vi "Autonomous Independent.vi"() -> ()   [LabVIEW 2016]
doc: "This VI is called when autonomous begins, and will automatically be terminated when autonomous ends. You can carry out timed or sensor driven robot movement independently without needing to return to the caller."
uses:
  <vilib>/Rock Robotics/WPI/Solenoid/WPI_SolenoidValue.ctl
  <vilib>/Rock Robotics/WPI/Utilities/WPI_GetSetVariantRefNum.vi
  <vilib>/Rock Robotics/Network Tables/NT Read String.vi
  <vilib>/Rock Robotics/Network Tables/NT Write Numeric Array.vi
  <vilib>/Rock Robotics/WPI/Solenoid/WPI_SolenoidSetEnum.vi
  SubSystems/Drive/Drive System.lvlib
  SubSystems/Intake/Intake.lvlib
  Vision/Vision Drive/Vision Drive.lvlib
  SubSystems/Path Track/Path Track.lvlib
panel:
  in  "Gear Auton Settings":T1(tab)=enum."Boiler Side Auton"
  in  "Center Gear Distance":dbl=81.0
  in  "First Turn Angle Hopper":dbl=60.0 caption="First Turn Angle"
  in  "First Drive Distance Hopper":dbl=95.0 caption="First Drive Distance"
  in  "Second Drive Distance Hopper":dbl=53.0 caption="Second Drive Distance"
  in  "Second Drive Distance":dbl=53.0
  in  "First Turn Angle":dbl=-60.0
  in  "First Drive Distance":dbl=95.0
  out "Distance (in) 2":dbl
  in  "Angle 2":dbl=30.0 format="%#_13g"
  in  "Distance (in)":dbl=-120.0 format="%#_13g"
  # "Distances:\n\n93.25\" to alignment line\n114.3\" to front of airship"
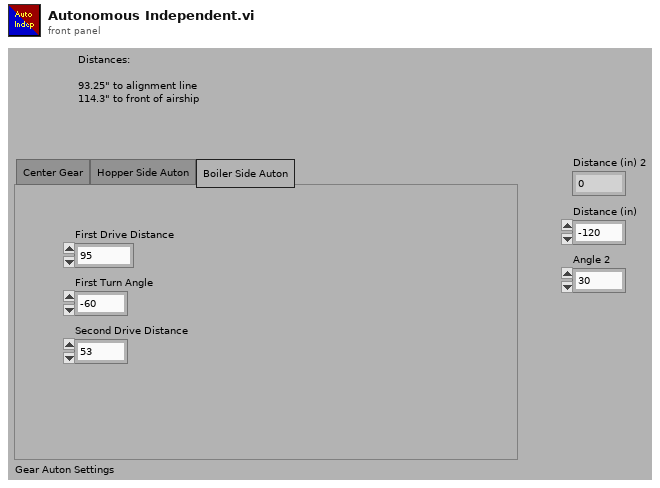
[diagram p1: front panel]
types:
  T1 = enum32{"Center Gear", "Hopper Side Auton", "Boiler Side Auton"}
  T2 = typedef "WPI_SolenoidValue.ctl" = enum16{"Off", "On", "Forward", "Reverse"}
  T3 = typedef "WPI_JoystickDevRef.ctl" = cluster{"Device":T4}
  T4 = typedef "WPI_JoystickDeviceEnum.ctl" = enum16{"USB 0", "USB 1", "USB 2", "USB 3", "USB 4", "USB 5"}
  T5 = typedef "WPI_SolenoidDevRef.ctl" = cluster{"DevStatus":errorcluster, "Pneumatics Control Module":u8, "Forward Solenoid Channel":T6, "Reverse Solenoid Channel":T6}
  T6 = typedef "WPI_SolenoidChannel.ctl" = enum8{"Solenoid 0", "Solenoid 1", "Solenoid 2", "Solenoid 3", "Solenoid 4", "Solenoid 5", "Solenoid 6", "Solenoid 7", "Invalid"}
  T7 = enum16{"Do Nothing", "Turn Up Field", "Turn to Boiler"}
  T8 = typedef "WPI_GyroDevRef.ctl" = cluster{"DevStatus":errorcluster, "Analog Channel":T9, "Offset":dbl, "Gain (VoltsPerDegree/Second)":dbl, "Gyro Type":enum16{"Analog", "XRS450"}, "Handle":i32, "SPI Bus":T10, "Device Found":bool, "Sample Rate":dbl, "Calibrate On Open":bool}
  T9 = typedef "FPGA_AIChannel.ctl" = enum8{"AI 0", "AI 1", "AI 2", "AI 3", "AI MXP 0", "AI MXP 1", "AI MXP 2", "AI MXP 3", "Invalid"}
  T10 = typedef "spi_bus.ctl" = enum16{"SPI On-Board, CS0", "SPI On-Board, CS1", "SPI On-Board, CS2", "SPI On-Board, CS3", "SPI MXP", "Invalid"}
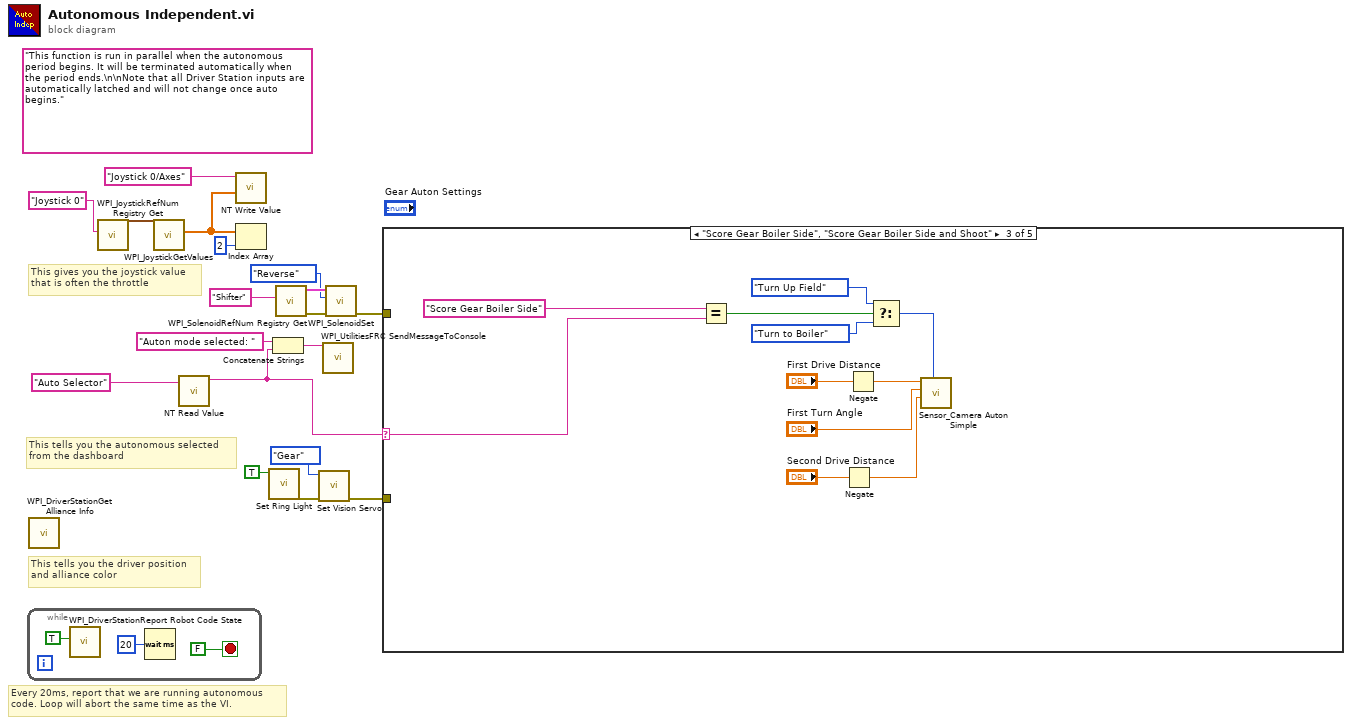
[diagram p0: block diagram]
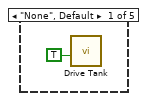
[diagram p2: hidden frame]
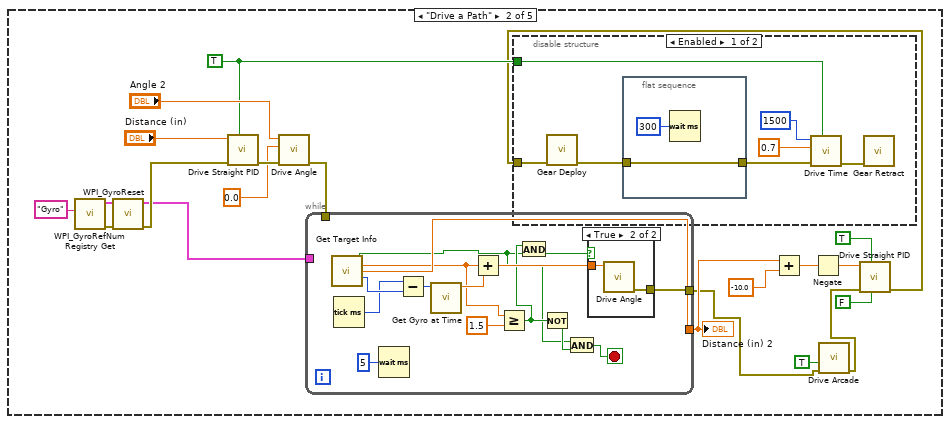
[diagram p3: hidden frame]
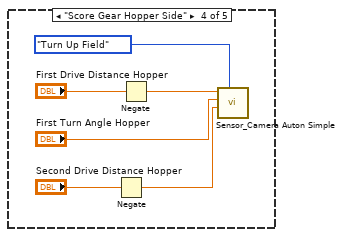
[diagram p6: hidden frame]
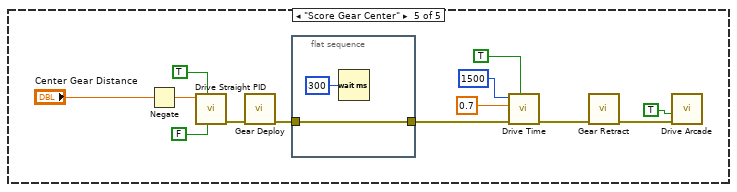
[diagram p7: hidden frame]
diagram:
  (unwired) "This function is run in parallel when the autonomous period begins. It will be terminated automatically when the period ends.\n\nNote that all Driver Station inputs are automatically latched and will not change once auto begins."
  # "This tells you the autonomous selected\nfrom the dashboard"
  # "Every 20ms, report that we are running autonomous\ncode. Loop will abort the same time as the VI."
  # "This gives you the joystick value\nthat is often the throttle"
  # "This tells you the driver position\nand alliance color"
  n1 = while {
    stop <- FALSE stop-if-true
    n2 = call <vilib>:"WPI_DriverStationReport Robot Code State.vi"("Autonomous"=TRUE) -> ()  [unwired: 10 in, 1 out]
    n3 = Wait (ms)(milliseconds to wait=u32 20) -> ()  [unwired: 1 out]
  }
  n4 = call <vilib>:"WPI_DriverStationGet Alliance Info.vi"() -> ()  [unwired: 12 out]
  n5 = call <vilib>:"WPI_JoystickRefNum Registry Get.vi"("refnum name"="Joystick 0") -> ("JoystickDevRef"=w17:T3)  [unwired: 1 in, 9 out]
  n6 = call <vilib>:"WPI_JoystickGetValues.vi"("JoystickDevRef"=w17) -> ("Axes"=w14:dbl[])  [unwired: 6 in, 4 out]
  n7 = call-poly <vilib>:"NT Read Value.vi"("Name"="Auto Selector") -> ("String"=w10:string)  [unwired: 9 in, 1 out]
  n8 = call-poly <vilib>:"NT Write Value.vi"("Numeric Array"=w14, "Name"="Joystick 0/Axes") -> ()  [unwired: 9 in, 1 out]
  n9 = Index Array(array=w14, index=2) -> ()  [unwired: 1 out]
  n10 = call "Set Ring Light.vi"("Light On? (F)"=TRUE) -> ("error out"=w7:errorcluster)  [unwired: 10 in]
  n11 = Concatenate Strings("Auton mode selected: " ("string"), w10) -> (w11:string)
  n12 = call <vilib>:"WPI_SolenoidRefNum Registry Get.vi"("refnum name"="Shifter") -> ("error out"=w4:errorcluster, "SolenoidDevRef"=w3:T5)  [unwired: 9 in]
  n13 = call "Set Vision Servo.vi"("error in"=w7, "Setting"=enum16{"Custom", "Boiler", "Gear"}."Gear") -> ("error out"=w6:errorcluster)  [unwired: 9 in]
  n14 = call <vilib>:"WPI_UtilitiesFRC SendMessageToConsole.vi"("Message"=w11) -> ()  [unwired: 14 in, 1 out]
  n15 = call-poly <vilib>:"WPI_SolenoidSet.vi"("error in (no error)"=w4, "Value"=WPI_SolenoidValue."Reverse", "SolenoidDevRef"=w3) -> ("error out"=w1:errorcluster)  [unwired: 7 in, 1 out]
  n16 = case shown="\"Score Gear Boiler Side\", \"Score Gear Boiler Side and Shoot\"" w10 {
    selector: w10 -> [_ _ w76 _ _]
    tunnel: w6 -> [_ _ _ _ _]
    tunnel: w1 -> [_ _ _ _ _]
    frame "None", Default {
      n17 = call "Drive Tank.vi"("Force? (F)"=TRUE) -> ()  [unwired: 10 in, 1 out]
    }
    frame "Drive a Path" {
      w41 = TRUE ("Wait for Completion? (F)")
      n18 = call <vilib>:"WPI_GyroRefNum Registry Get.vi"("refnum name"="Gyro") -> ("error out"=w39:errorcluster, "GyroDevRef"=w38:T8)  [unwired: 9 in]
      n19 = call <vilib>:"WPI_GyroReset.vi"("error in"=w39, "GyroDevRef"=w38) -> ("error out"=w36:errorcluster, "GyroDevRef"=w34:T8)  [unwired: 8 in]
      n20 = call "Drive Straight PID.vi"("Wait for Completion? (F)"=w41, "error in"=w36, "Distance (in)"="Distance (in)") -> ("error out"=w43:errorcluster)  [unwired: 8 in]
      n21 = call "Drive Angle.vi"("error in"=w43, "Drive Magnitude"=0.0, "Angle"="Angle 2") -> ("error out"=w35:errorcluster)  [unwired: 8 in]
      n22 = while {
        tunnel: w35 -> [_]
        tunnel: w34 -> [_]
        tunnel: [w52] -> w32
        tunnel: [w47] -> w26
        stop <- w49 stop-if-true
        n23 = call "Get Target Info.vi"() -> ("Target Found?"=w48:bool, "Angle (deg)"=w51:dbl, "Distance (in)"=w52:dbl, "timestamp"=w46:u32)  [unwired: 11 in, 1 out]
        n24 = Tick Count (ms)() -> (millisecond timer value=w44:u32)
        n25 = Wait (ms)(milliseconds to wait=u32 5) -> ()  [unwired: 1 out]
        n26 = Subtract(x=w44, y=w46) -> (x-y=w45:u32)
        n27 = call "Get Gyro at Time.vi"("Get ms ago"=w45) -> ("Angle"=w57:dbl)  [unwired: 9 in, 1 out]
        n28 = Add(x=w51, y=w57) -> (x+y=w56:dbl)
        n29 = Greater Or Equal?(x=w51, y=1.5) -> (x >= y?=w53:bool)
        n30 = And(x=w53, y=w48) -> (x .and. y?=w54:bool)
        n31 = Not(x=w53) -> (.not. x?=w50:bool)
        n32 = And(x=w48, y=w50) -> (x .and. y?=w49:bool)
        n33 = case shown="True" w54 {
          tunnel: w56 -> [_ w60]
          tunnel: [_ w59] -> w47
          frame False {
          }
          frame True {
            n34 = call "Drive Angle.vi"("Angle"=w60) -> ("error out"=w59:errorcluster)  [unwired: 10 in]
          }
        }
      }
      "Distance (in) 2" <- w32
      n35 = Add(x=w32, y=-10.0 ("Peg dist")) -> (x+y=w33:dbl)
      n36 = Negate(x=w33) -> (-x=w24:dbl)
      n37 = call "Drive Arcade.vi"("error in"=w26, "Force? (F)"=TRUE) -> ("error out"=w25:errorcluster)  [unwired: 9 in]
      n38 = call "Drive Straight PID.vi"("Force? (F)"=FALSE, "Wait for Completion? (F)"=TRUE, "error in"=w25, "Distance (in)"=w24) -> ("error out"=w28:errorcluster)  [unwired: 7 in]
      n39 = disable-structure shown="Enabled" {
        disable-tunnel: w41 -> [w65 _]
        disable-tunnel: w28 -> [w64 _]
        frame Enabled {
          n40 = call "Gear Deploy.vi"("error in"=w64) -> ("error out"=w63:errorcluster)  [unwired: 10 in]
          n41 = flat-sequence {
            tunnel: w63 -> [w69]
            tunnel: [w69] -> w62
            frame #0 {
              n42 = Wait (ms)(milliseconds to wait=u32 300) -> ()  [unwired: 1 out]
            }
          }
          n43 = call "Drive Time.vi"("Wait for Completion? (F)"=w65, "error in"=w62, "Y Axis"=0.7, "Time (ms)"=u32 1500) -> ("error out"=w61:errorcluster)  [unwired: 7 in]
          n44 = call "Gear Retract.vi"("error in"=w61) -> ()  [unwired: 10 in, 1 out]
        }
        frame Disabled {
        }
      }
    }
    frame "Score Gear Boiler Side", "Score Gear Boiler Side and Shoot" {
      n45 = Equal?(x="Score Gear Boiler Side" ("refnum name"), y=w76) -> (x = y?=w75:bool)
      n46 = Negate(x="Second Drive Distance") -> (-x=w70:dbl)
      n47 = Negate(x="First Drive Distance") -> (-x=w71:dbl)
      n48 = Select(t=T7."Turn Up Field" ("Final Task"), s=w75, f=T7."Turn to Boiler" ("Final Task")) -> (s? t:f=w74:T7)
      n49 = call "Sensor_Camera Auton Simple.vi"("Final Task"=w74, "Second Drive Distance"=w70, "First Turn Angle"="First Turn Angle", "First Drive Distance"=w71) -> ()  [unwired: 7 in, 1 out]
    }
    frame "Score Gear Hopper Side" {
      n50 = Negate(x="Second Drive Distance Hopper") -> (-x=w81:dbl)
      n51 = Negate(x="First Drive Distance Hopper") -> (-x=w82:dbl)
      n52 = call "Sensor_Camera Auton Simple.vi"("Final Task"=T7."Turn Up Field", "Second Drive Distance"=w81, "First Turn Angle"="First Turn Angle Hopper", "First Drive Distance"=w82) -> ()  [unwired: 7 in, 1 out]
    }
    frame "Score Gear Center" {
      n53 = Negate(x="Center Gear Distance") -> (-x=w87:dbl)
      n54 = call "Drive Straight PID.vi"("Force? (F)"=FALSE, "Wait for Completion? (F)"=TRUE, "Distance (in)"=w87) -> ("error out"=w97:errorcluster)  [unwired: 8 in]
      n55 = call "Gear Deploy.vi"("error in"=w97) -> ("error out"=w98:errorcluster)  [unwired: 10 in]
      n56 = flat-sequence {
        tunnel: w98 -> [w101]
        tunnel: [w101] -> w90
        frame #0 {
          n57 = Wait (ms)(milliseconds to wait=u32 300) -> ()  [unwired: 1 out]
        }
      }
      n58 = call "Drive Time.vi"("Wait for Completion? (F)"=TRUE, "error in"=w90, "Y Axis"=0.7, "Time (ms)"=u32 1500) -> ("error out"=w96:errorcluster)  [unwired: 7 in]
      n59 = call "Gear Retract.vi"("error in"=w96) -> ("error out"=w92:errorcluster)  [unwired: 10 in]
      n60 = call "Drive Arcade.vi"("error in"=w92, "Force? (F)"=TRUE) -> ()  [unwired: 9 in, 1 out]
    }
  }
